vi "Robot Global Data.vi"() -> ()   [LabVIEW 2015]
doc: "This global VI can contain as many global variables as you need. Place a control on the panel, give it a good name. To read or write to it from a VI, drag the icon to the diagram of that VI. You can also drag from the project. Click on the node to change which global you access. You shouldn't have multiple locations writing to a global or it will cause a race-condition."
uses:
  <vilib>/Rock Robotics/WPI/DriverStation/WPI_DriverStationRobotMode2.ctl
  <vilib>/vision/Image Controls.llb/IMAQ Image.ctl
panel:
  in  "Vision Processing Enabled":bool
  in  "Vision Processing Notifier":refnum<notifier>
  in  "intake":bool
  in  "camOn":bool
  out "start degree":dbl
  in  "Turn 90":refnum<k4>
  in  "Ball Intake":refnum<k4>
  in  "lightOn":bool
  out "Encoder Limit":bool
  in  "Shoot Occurrence":refnum<k4>
  in  "Camera":enum16{"Camera 1", "Camera 2"}(ring)
  out "CancelTurn":bool
  out "RotateRight":bool
  out "Rotate":bool
  in  "Robot Mode":T1
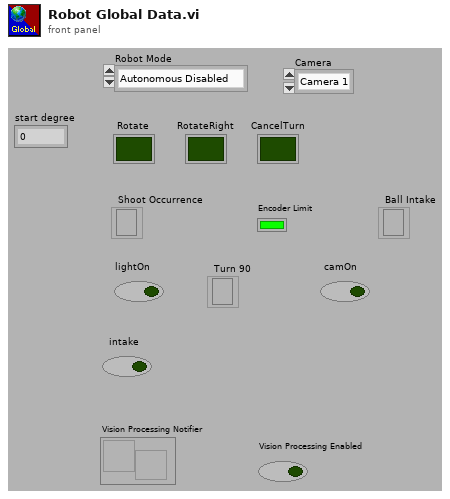
[diagram p1: front panel]
types:
  T1 = typedef "WPI_DriverStationRobotMode2.ctl" = enum16{"Autonomous Disabled", "Autonomous Enabled", "Teleop Disabled", "Teleop Enabled", "Disconnected", "Finish", "Test Disabled", "Test Enabled", "Emergency Stopped"}
diagram:
